vi "Build DashBoard Data.vi"(11 "Dashboard Enables":T3={"Analog Module 1"=[TRUE, TRUE, TRUE, TRUE, TRUE, TRUE, TRUE, TRUE], "Analog Module 2"=[FALSE, FALSE, FALSE, FALSE, FALSE, FALSE, FALSE, FALSE], "Digital Module 1"=TRUE, "Digital Module 2"=FALSE, "Solenoid Module"=TRUE}) -> ()   [LabVIEW 2011]
doc: "This VI builds data and sends it back to the dashboard PC program. By default it sends back the raw values for the first analog, digital, and solenoid module. Modify it to send back the data you want to view. Consider adding higher level data to the Dashboard Datatype.ctl and to this VI. Then update the Dashboard to display the data however you like.\n\nThis software is licensed. Open the labview\\readme\\WPI Robotics Library Open Source License.txt file for more information."
uses:
  DashboardEnable.ctl
  Dashboard Datatype.ctl
  <vilib>/Rock Robotics/WPI/DriverStation/WPI_DriverStationDigitalData.ctl
  Robot Global Data.vi
panel:
  out "Dashboard Data":T1
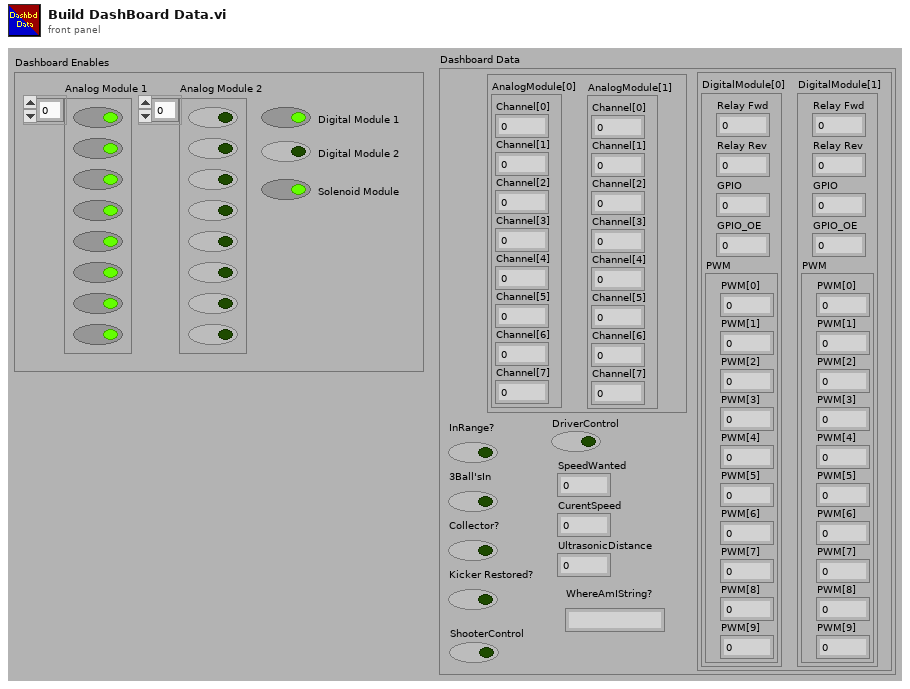
[diagram p1: front panel]
types:
  T1 = typedef "Dashboard Datatype.ctl" = cluster{cluster{"AnalogModule[0]":cluster{"Channel[0]":sgl, "Channel[1]":sgl, "Channel[2]":sgl, "Channel[3]":sgl, "Channel[4]":sgl, "Channel[5]":sgl, "Channel[6]":sgl, "Channel[7]":sgl}, "AnalogModule[1]":cluster{"Channel[0]":sgl, "Channel[1]":sgl, "Channel[2]":sgl, "Channel[3]":sgl, "Channel[4]":sgl, "Channel[5]":sgl, "Channel[6]":sgl, "Channel[7]":sgl}}, cluster{"DigitalModule[0]":T2, "DigitalModule[1]":T2}, "SpeedWanted":dbl, "CurentSpeed":dbl, "UltrasonicDistance":dbl, "3Ball'sIn":bool, "Collector?":bool, "Kicker Restored?":bool, "InRange?":bool, "DriverControl":bool, "ShooterControl":bool, "WhereAmIString?":string}
  T2 = typedef "WPI_DriverStationDigitalData.ctl" = cluster{"Relay Fwd":u8, "Relay Rev":u8, "GPIO":u16, "GPIO_OE":u16, "PWM":cluster{"PWM[0]":u8, "PWM[1]":u8, "PWM[2]":u8, "PWM[3]":u8, "PWM[4]":u8, "PWM[5]":u8, "PWM[6]":u8, "PWM[7]":u8, "PWM[8]":u8, "PWM[9]":u8}}
  T3 = typedef "DashboardEnable.ctl" = cluster{"Analog Module 1":bool[], "Analog Module 2":bool[], "Digital Module 1":bool, "Digital Module 2":bool, "Solenoid Module":bool}
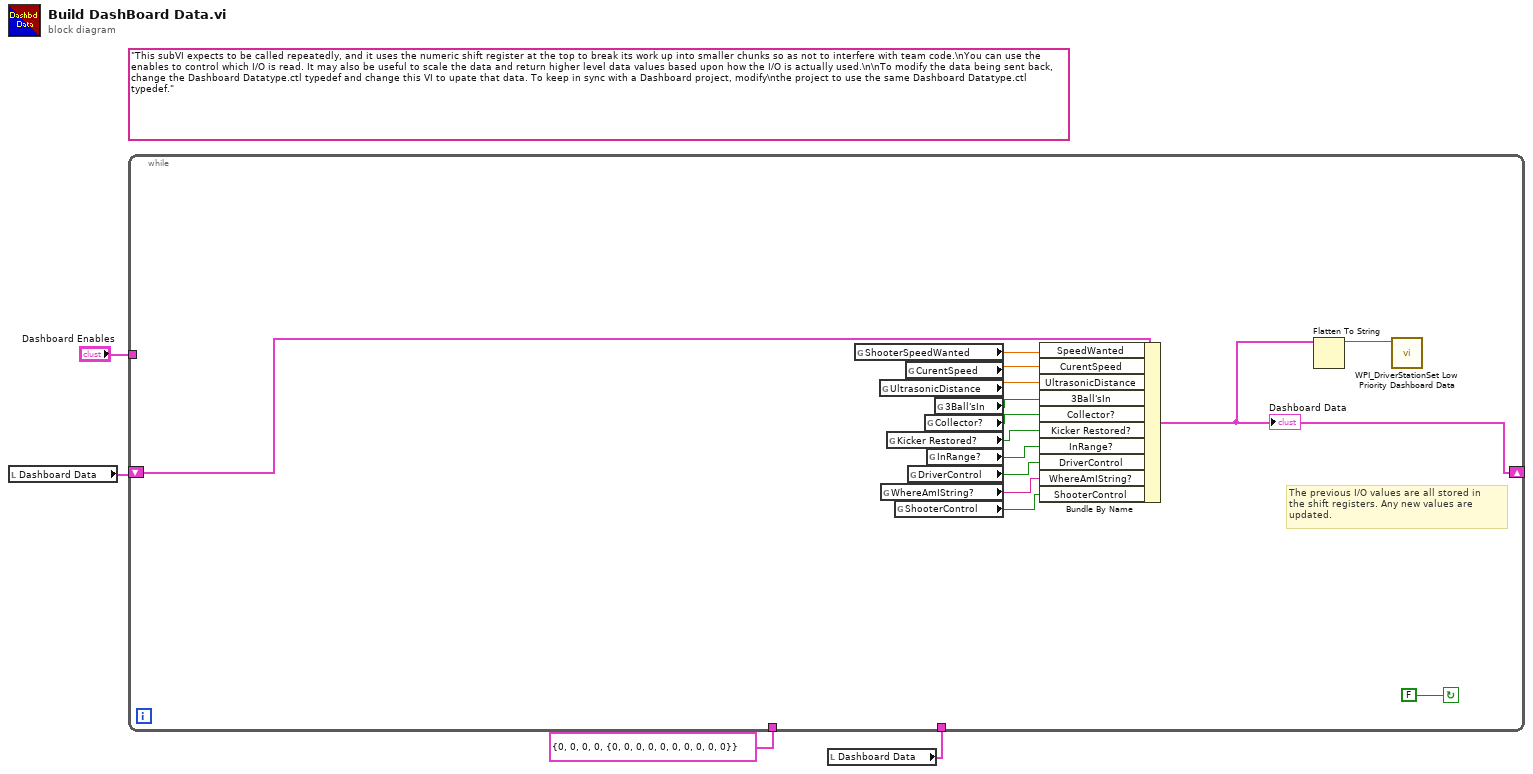
[diagram p0: block diagram]
diagram:
  (unwired) "This subVI expects to be called repeatedly, and it uses the numeric shift register at the top to break its work up into smaller chunks so as not to interfere with team code.\nYou can use the enables to control which I/O is read. It may also be useful to scale the data and return higher level data values based upon how the I/O is actually used.\n\nTo modify the data being sent back, change the Dashboard Datatype.ctl typedef and change this VI to upate that data. To keep in sync with a Dashboard project, modify\nthe project to use the same Dashboard Datatype.ctl typedef."
  n1 = local read "Dashboard Data"() -> (w1:T1)
  n2 = local read "Dashboard Data"() -> (w3:T1)
  n3 = while {
    shift-right: [w11] -> _
    shift-left: w1 -> [w10]
    tunnel: T2 {"Relay Fwd"=0, "Relay Rev"=0, "GPIO"=0, "GPIO_OE"=0, "PWM"={"PWM[0]"=0, "PWM[1]"=0, "PWM[2]"=0, "PWM[3]"=0, "PWM[4]"=0, "PWM[5]"=0, "PWM[6]"=0, "PWM[7]"=0, "PWM[8]"=0, "PWM[9]"=0}} ("DigitalModule[1]") -> [_]
    tunnel: w3 -> [_]
    tunnel: "Dashboard Enables" -> [_]
    stop <- FALSE continue-if-true
    # "The previous I/O values are all stored in\nthe shift registers. Any new values are\nupdated."
    n4 = global read "Robot Global Data.vi" "ShooterSpeedWanted"() -> (w17:dbl)
    n5 = global read "Robot Global Data.vi" "UltrasonicDistance"() -> (w15:dbl)
    n6 = global read "Robot Global Data.vi" "WhereAmIString?"() -> (w6:string)
    n7 = global read "Robot Global Data.vi" "Kicker Restored?"() -> (w13:bool)
    n8 = global read "Robot Global Data.vi" "ShooterControl"() -> (w5:bool)
    n9 = global read "Robot Global Data.vi" "CurentSpeed"() -> (w16:dbl)
    n10 = global read "Robot Global Data.vi" "DriverControl"() -> (w7:bool)
    n11 = global read "Robot Global Data.vi" "Collector?"() -> (w14:bool)
    n12 = global read "Robot Global Data.vi" "InRange?"() -> (w12:bool)
    n13 = global read "Robot Global Data.vi" "3Ball'sIn"() -> (w9:bool)
    n14 = Bundle By Name(cluster=w10, "SpeedWanted"=w17, "CurentSpeed"=w16, "UltrasonicDistance"=w15, "3Ball'sIn"=w9, "Collector?"=w14, "Kicker Restored?"=w13, "InRange?"=w12, "DriverControl"=w7, "WhereAmIString?"=w6, "ShooterControl"=w5) -> (w11:T1)
    "Dashboard Data" <- w11
    n15 = Flatten To String(anything=w11) -> (data string=w8:string)  [unwired: 1 in, 4 out]
    n16 = call <vilib>:"WPI_DriverStationSet Low Priority Dashboard Data.vi"("User Data"=w8) -> ()  [unwired: 1 in, 10 out]
  }
